vi "TestPanelValueChange.vi"() -> ()   [LabVIEW 2020]
uses:
  Test.Maui 2.0.Panels/Test.Maui 2.0.Panels.lvclass
panel:
  out "error out":errorcluster
  in  "error in":errorcluster
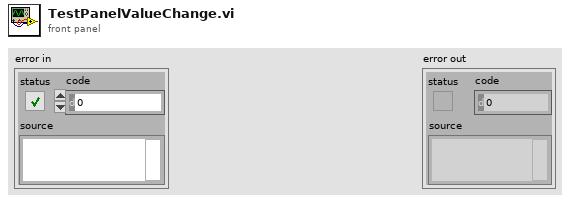
[diagram p1: front panel]
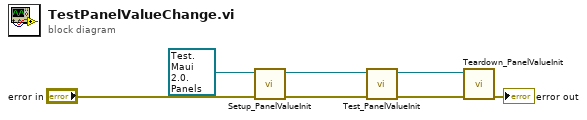
[diagram p0: block diagram]
diagram:
  n1 = call "Setup_PanelValueInit.vi"("error in (no error)"="error in", "Test.Maui 2.0.Panels in"=refnum<class "Test.Maui 2.0.Panels.lvclass"> refnum ("Test.Maui 2.0.Panels.lvclass")) -> ("error out"=w5:errorcluster, "Test.Maui 2.0.Panels out"=w6:refnum<class "Test.Maui 2.0.Panels.lvclass">)  [unwired: 8 in]
  n2 = call "Test_PanelValueInit.vi"("error in (no error)"=w5, "Test.Maui 2.0.Panels in"=w6) -> ("error out"=w3:errorcluster, "Test.Maui 2.0.Panels out"=w4:refnum<class "Test.Maui 2.0.Panels.lvclass">)  [unwired: 8 in]
  n3 = call "Teardown_PanelValueInit.vi"("error in (no error)"=w3, "Test.Maui 2.0.Panels in"=w4) -> ("error out"=→"error out":errorcluster)  [unwired: 8 in, 1 out]
